vi "DHE_get_autoclear.vi"(0 "fd in":i32, 11 "error in (no error)":errorcluster) -> (4 "fd out":i32, 6 "autoclear":bool, 15 "error out":errorcluster)   [LabVIEW 2016]
doc: "This VI closes the I/O interface with the instrument."
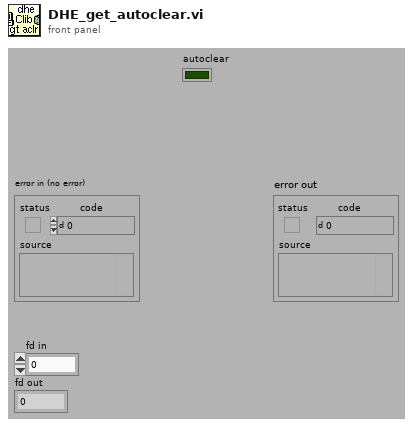
[diagram p1: front panel]
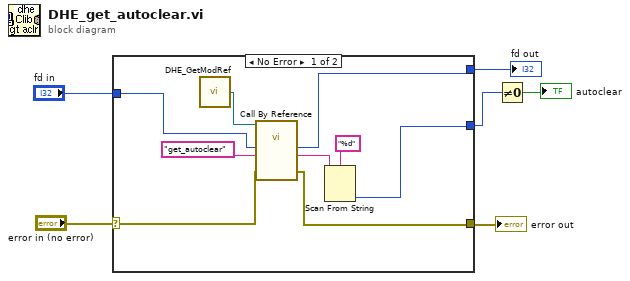
[diagram p0: block diagram]
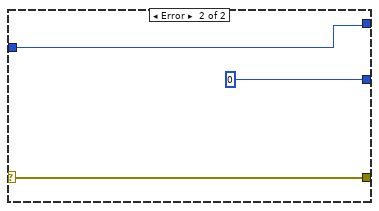
[diagram p2: hidden frame]
diagram:
  n1 = case shown="No Error" "error in (no error)" {
    selector: "error in (no error)" -> [w9 w18]
    tunnel: [w8 w18] -> w6
    tunnel: [w7 0 ("sequence")] -> w4
    tunnel: "fd in" -> [w11 w16]
    tunnel: [w10 w16] -> w1
    frame No Error {
      n2 = call "DHE_GetModRef.vi"() -> ("DHE_ModRef"=w15:refnum<vi>)  [unwired: 9 out]
      n3 = call-by-ref "?"(reference=w15, "error in (no error)"=w9, "function"="get_autoclear", "fd in"=w11) -> ("error out"=w8:errorcluster, "str result"=w13:string, "fd out"=w10:i32)  [unwired: 6 in, 3 out]
      n4 = Scan From String(format string="%d", input string=w13) -> (output 1=w7:i32)  [unwired: 2 in, 4 out]
    }
    frame Error {
    }
  }
  "error out" <- w6
  "fd out" <- w1
  n5 = Not Equal To 0?(x=w4) -> (x != 0?=→"autoclear":bool)
